vi "Get Coverage Percentage.vi"(8 "error in (no error)":errorcluster, 10 "VI Path":path, 11 "CodeCoverage in":refnum<class "CodeCoverage.lvclass">) -> (0 "error out":errorcluster, 2 "Coverage Percentage":dbl, 3 "CodeCoverage out":refnum<class "CodeCoverage.lvclass">)   [LabVIEW 2017, in "CodeCoverage.lvclass"]
doc: "Returns the code coverage percentage for a given VI."
uses:
  CodeCoverage.lvclass
  CodeCoverage.lvclass/CodeCoverage.ctl
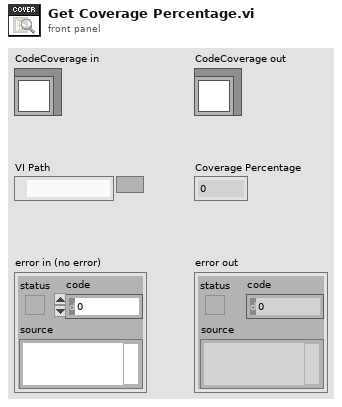
[diagram p1: front panel]
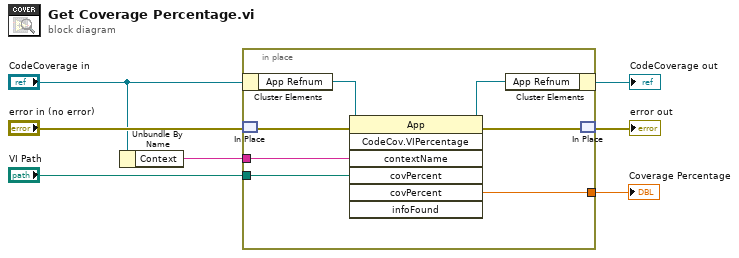
[diagram p0: block diagram]
diagram:
  n1 = Unbundle By Name("CodeCoverage in") -> ("Context"=w5:string)
  n2 = in-place {
    in-place-border: "VI Path" -> [w14]
    in-place-border: [w13] -> w6
    in-place-border: w5 -> [w12]
    n3 = in-place-cluster #1("CodeCoverage in") -> ("App Refnum"=w9:refnum<vi>)
    n4 = in-place-match #2("error in (no error)") -> (w11:errorcluster)
    n5 = invoke class="App" method="CodeCov.VIPercentage"(reference=w9, error in=w11, "contextName"=w12, "covPercent"=w14) -> (reference out=w8:refnum<vi>, error out=w10:errorcluster, "covPercent"=w13:dbl)  [unwired: 3 in, 4 out]
    n6 = in-place-cluster #1("App Refnum"=w8) -> (→"CodeCoverage out":refnum<class "CodeCoverage.lvclass">)
    n7 = in-place-match #2(w10) -> (→"error out":errorcluster)
  }
  "Coverage Percentage" <- w6
